vi "Overview Cursor Grab.vi"(8 "error in (no error)":errorcluster, 11 "XYGraphOverview in":refnum<class "XYGraphOverview.lvclass">) -> (0 "error out":errorcluster, 3 "XYGraphOverview out":refnum<class "XYGraphOverview.lvclass">)   [LabVIEW 2020, in "XYGraphOverview.lvlib" / "XYGraphOverview.lvclass"]
uses:
  XYGraphOverview.lvclass
  XYGraphOverview.lvclass/XYGraphOverview.ctl
  Read Block Color.vi
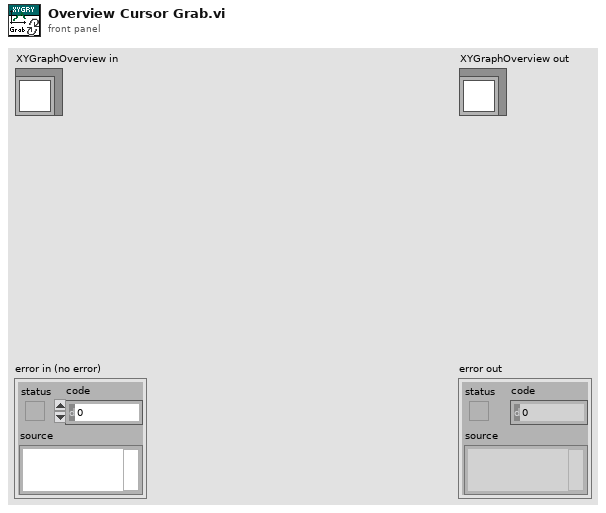
[diagram p1: front panel]
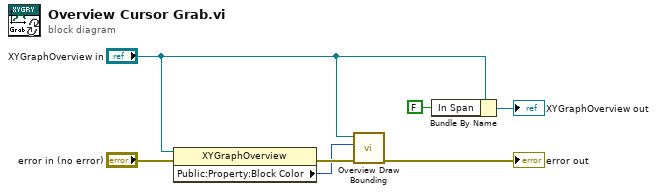
[diagram p0: block diagram]
diagram:
  n1 = property class="XYGraphOverview"(reference="XYGraphOverview in", error in="error in (no error)") -> (error out=w6:errorcluster, "Public:Property:Block Color"=w5:u32)  [unwired: 1 out]
  n2 = call "Overview Draw Bounding.vi"("error in (no error)"=w6, "Color"=w5, "XYGraphOverview in"="XYGraphOverview in") -> ("error out"=→"error out":errorcluster)  [unwired: 7 in, 1 out]
  n3 = Bundle By Name(cluster="XYGraphOverview in", "In Span"=FALSE) -> (→"XYGraphOverview out":refnum<class "XYGraphOverview.lvclass">)
